vi "LabviewTest.vi"() -> ()   [LabVIEW 2018]
uses:
  Program Files (x86)/National Instruments/LabVIEW 2018/examples/Connectivity/Python/support/PythonVersionsEnum.ctl
  PythonConfigGlobal.vi
panel:
  in  "탭 컨트롤":T1(tab)
  in  "array":dbl[](array[numeric])
  out "mean":dbl
  out "variance":dbl
  out "standard deviation":dbl
  in  "error type":u16(ring) items=["RMSE", "MAE", "RTE", "Approximate E", "3", "2", "1"]
  in  "targets":dbl[](array[numeric])
  in  "predictions":dbl[](array[numeric])
  out "ans array":dbl[](array[numeric])
  out "ans":dbl
  in  "x":dbl[][](array[numeric])
  out "covariance matrix V":dbl[][](array[numeric])
  out "mean vector":dbl[](array[numeric]) caption="평균 벡터"
  in  "y":dbl[](array[numeric])
  in  "x":dbl[](array[numeric])
  out "correlation coefficient r":dbl caption="상관 계수 r" format="%.7g"
  out "r^2":dbl format="%.7g"
  in  "python version":T2=enum."3.6"
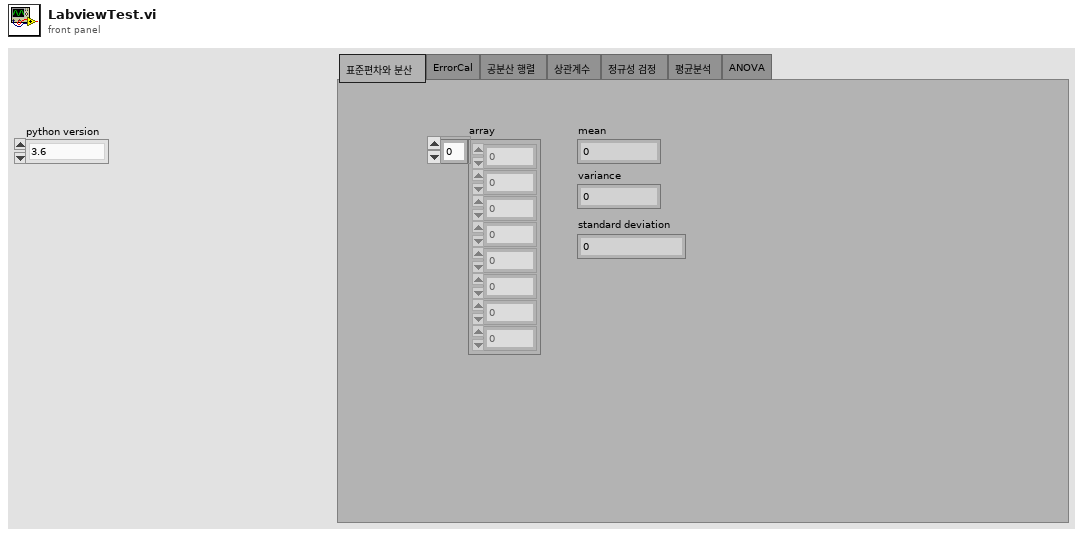
[diagram p1: front panel]
types:
  T1 = enum32{"표준편차와 분산", "ErrorCal", "공분산 행렬", "상관계수", "정규성 검정", "평균분석", "ANOVA"}
  T2 = typedef "PythonVersionsEnum.ctl" = enum16{"2.7", "3.6"}
  T3 = cluster{"session out":refnum<k35>, "appended path":path}
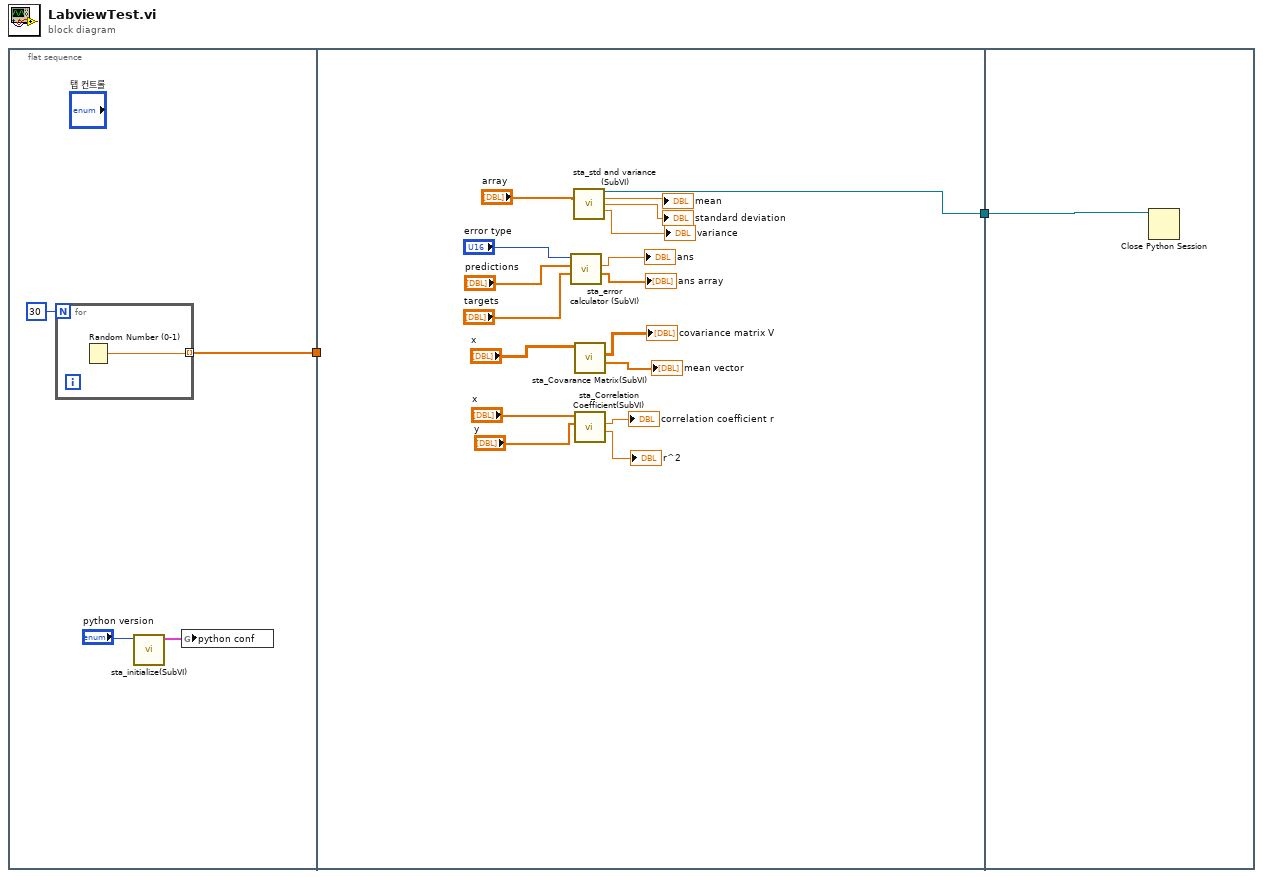
[diagram p0: block diagram]
diagram:
  n1 = flat-sequence {
    tunnel: [w3] -> w1
    tunnel: [w24] -> w2
    tunnel: w1 -> [_]
    tunnel: w2 -> [w25]
    frame #0 {
      n2 = for {
        N: 30 -> [_]
        tunnel: [w7] -> w3 mode=indexing
        n3 = Random Number (0-1)() -> (number: 0 to 1=w7:dbl)
      }
      n4 = call "sta_initialize(SubVI).vi"("python version"="python version") -> ("클러스터"=w5:T3)  [unwired: 10 in]
      n5 = global write "PythonConfigGlobal.vi" "python conf"(w5) -> ()
    }
    frame #1 {
      n6 = call "sta_error calculator (SubVI).vi"("targets"="targets", "predictions"="predictions", "error type"="error type") -> ("ans array"=→"ans array":dbl[], "ans"=→"ans":dbl)  [unwired: 5 in, 2 out]
      n7 = call "sta_std and variance (SubVI).vi"("array"="array") -> ("참조 번호 출력"=w24:refnum<k35>, "mean"=→"mean":dbl, "standard deviation"=→"standard deviation":dbl, "variance"=→"variance":dbl)  [unwired: 10 in, 1 out]
      n8 = call "sta_Covarance Matrix(SubVI).vi"("x"="x") -> ("mean vector"=→"mean vector":dbl[], "covariance matrix V"=→"covariance matrix V":dbl[][])  [unwired: 7 in, 2 out]
      n9 = call "sta_Correlation Coefficient(SubVI).vi"("y"="y", "x"="x") -> ("r^2"=→"r^2":dbl, "correlation coefficient r"=→"correlation coefficient r":dbl)  [unwired: 6 in, 2 out]
    }
    frame #2 {
      n10 = Close Python Session(session in=w25) -> ()  [unwired: 1 in, 1 out]
    }
  }
